vi "Power Test.vi"(9 "TDMS File Path In":string, 10 "Current (A)":dbl, 11 "Voltage (V)":dbl) -> (1 "TDMS File Path":string, 3 "Power (W)":dbl)   [LabVIEW 2019]
panel:
  out "Power Loss":dbl
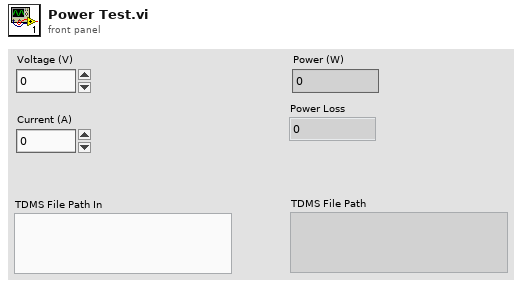
[diagram p1: front panel]
types:
  T1 = enum16{"open", "open or create", "create or replace", "create", "open (read-only)"}
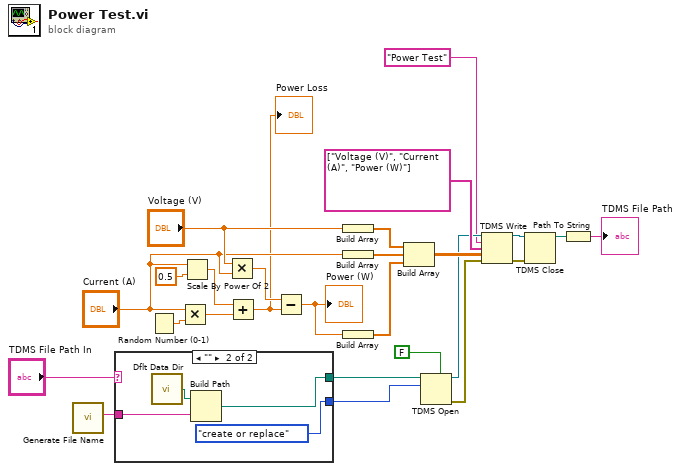
[diagram p0: block diagram]
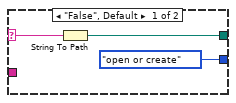
[diagram p2: hidden frame]
diagram:
  n1 = call "Generate File Name.vi"() -> ("file name"=w14:string)  [unwired: 9 in, 1 out]
  n2 = case shown="\"\"" "TDMS File Path In" {
    selector: "TDMS File Path In" -> [w28 _]
    tunnel: [T1."open or create" ("operation (0:open)") T1."create or replace" ("operation (0:open)")] -> w19
    tunnel: [w27 w31] -> w18
    tunnel: w14 -> [_ w30]
    frame "False", Default {
      n3 = String To Path(string=w28) -> (path=w27:path)
    }
    frame "" {
      n4 = call "Dflt Data Dir.vi"() -> ("App:Default Data Directory"=w33:path)
      n5 = Build Path(base path=w33, name or relative path=w30) -> (appended path=w31:path)
    }
  }
  n6 = Random Number (0-1)() -> (number: 0 to 1=w5:dbl)
  n7 = Multiply(x="Current (A)", y=w5) -> (x*y=w4:dbl)
  n8 = Scale By Power Of 2(n="Current (A)", x=0.5 ("y")) -> (x*2^n=w3:dbl)
  n9 = Multiply(x="Voltage (V)", y="Current (A)") -> (x*y=w8:dbl)
  n10 = Add(x=w3, y=w4) -> (x+y=w2:dbl)
  "Power Loss" <- w2
  n11 = Subtract(x=w8, y=w2) -> (x-y=w9:dbl)
  "Power (W)" <- w9
  n12 = Build Array("Voltage (V)") -> (w12:dbl[])
  n13 = Build Array("Current (A)") -> (w11:dbl[])
  n14 = Build Array(w9) -> (w10:dbl[])
  n15 = Build Array(w12, w11, w10) -> (w21:dbl[][])
  n16 = TDMS Open(5:FALSE ("create index file? (T)"), 10:w19, 11:w18) -> (0:w17:errorcluster, 3:w16:refnum<k34>)  [unwired: 4 in]
  n17 = TDMS Write(0:w16, 5:"Power Test" ("group name in (Untitled)"), 7:string[] ["Voltage (V)", "Current (A)", "Power (W)"] ("channel name(s) in (Untitled)"), 9:w21, 11:w17) -> (4:w26:refnum<k34>, 15:w25:errorcluster)  [unwired: 1 in, 2 out]
  n18 = TDMS Close(8:w25, 11:w26) -> (3:w23:path)  [unwired: 1 out]
  n19 = Path To String(path=w23) -> (string=→"TDMS File Path":string)
